vi "FPGA Reference FG.vi"() -> (3 "FPGA VI Reference Out":T1)   [LabVIEW 2013]
uses:
  FPGA_Reference.ctl
  <vilib>/userdefined/High Color/nirio_resource_hc.ctl
  <vilib>/FPGAPlugInAG/PCIe-1473R-LX110/niLvFpga_Open_PCIe-1473R-LX110.vi
  <vilib>/rvi/interface/nirviOpenFPGA/nirviOpenFPGA.xnode
  FPGA Bitfiles/WBA256SectorsSim_FPGATarget.lvbitx
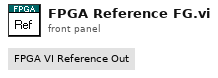
[diagram p1: front panel]
types:
  T1 = typedef "FPGA_Reference.ctl" = refnum<k20>
  T2 = typedef "nirio_resource_hc.ctl" = tag
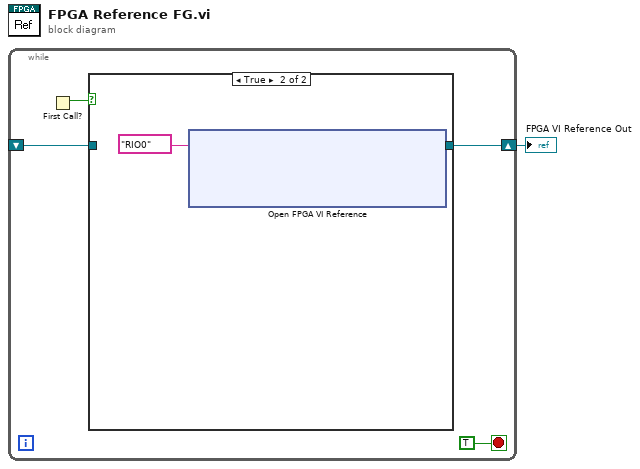
[diagram p0: block diagram]
diagram:
  n1 = while {
    shift-right: [w3] -> w1
    shift-left: _ -> [w2]
    stop <- TRUE stop-if-true
    n2 = First Call?() -> (First Call?: T/F=w5:bool)
    n3 = case shown="True" w5 {
      tunnel: [w6 w7] -> w3
      tunnel: w2 -> [w6 _]
      frame False {
      }
      frame True {
        n4 = xnode "Open FPGA VI Reference"("resource name"=T2 "RIO0") -> ("FPGA VI Reference Out"=w7:T1)  [unwired: 1 in, 1 out]
      }
    }
  }
  "FPGA VI Reference Out" <- w1
